vi "Reduce Motor Torque.vi"(4 "Delay Period (0ms)":i32 min=0 max=60000, 5 "error in (no error)":errorcluster, 6 "Motor Current Reduction (0%)":dbl min=0.0 max=100.0 format="%#.4g", 7 "Axis (1)":i32=1 min=1 max=3, 8 "VISA resource name":refnum<visa-resource-name>) -> (0 "error out":errorcluster, 3 "VISA resource name out":refnum<visa-resource-name>)   [LabVIEW 2019, in "Newport ESP301.lvlib"]
doc: "This command automatically reduces the specified step motor’s current (i.e., torque) output to the requested percentage <B>Motor Current Reduction (0%)</B> after motion has stopped and the specified time <B>Delay Period (0ms)</B> has expired. The purpose of this command is to help reduce the motor heating typically generated by stepper motors.\n<B>NOTE:</B> This command does not affect DC servo motors and pulse stepper motors."
uses:
  Newport ESP301.lvlib
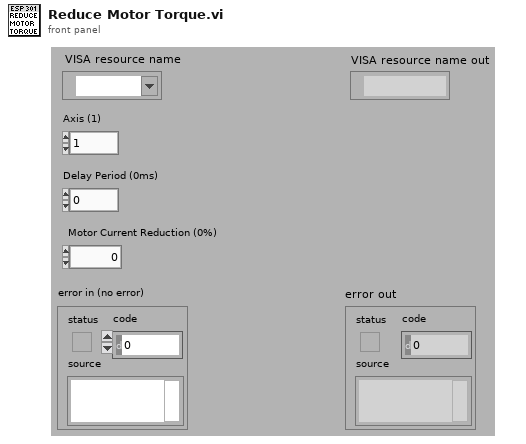
[diagram p1: front panel]
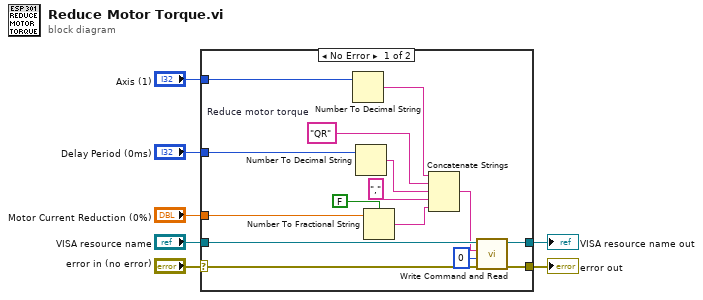
[diagram p0: block diagram]
diagram:
  n1 = case shown="No Error" "error in (no error)" {
    selector: "error in (no error)" -> [w21 w24]
    tunnel: [w20 w24] -> w7
    tunnel: "VISA resource name" -> [w22 w23]
    tunnel: [w19 w23] -> w6
    tunnel: "Axis (1)" -> [w16 _]
    tunnel: "Delay Period (0ms)" -> [w13 _]
    tunnel: "Motor Current Reduction (0%)" -> [w10 _]
    frame No Error {
      w17 = "QR"  # Reduce motor torque
      n2 = Number To Decimal String(number=w16) -> (decimal integer string=w18:string)  [unwired: 1 out]
      n3 = Number To Decimal String(number=w13) -> (decimal integer string=w12:string)  [unwired: 1 out]
      n4 = Number To Fractional String(use system decimal point (T)=FALSE ("utiliser le séparateur décimal du système (V)"), number=w10) -> (F-format string=w9:string)  [unwired: 2 in]
      n5 = Concatenate Strings(w18, w17, w12, "," ("Assign DIO Bits to Inhibit Motion"), w9) -> (w15:string)
      n6 = call "Write Command and Read.vi"("error in (no error)"=w21, "Bytes to read (100)"=u32 0, "Command"=w15, "VISA resource name"=w22) -> ("error out"=w20:errorcluster, "VISA resource name out"=w19:refnum<visa-resource-name>)  [unwired: 1 in, 3 out]
    }
    frame Error {
    }
  }
  "error out" <- w7
  "VISA resource name out" <- w6
